vi "DoOperationDynamicDispatchMethod.vi"(8 "error in (no error)":errorcluster, 11 "SimpleArithmetic in":refnum<class "SimpleArithmetic.lvclass">) -> (0 "error out":errorcluster, 3 "SimpleArithmetic out":refnum<class "SimpleArithmetic.lvclass">)   [LabVIEW 2010, in "SimpleArithmetic.lvclass"]
uses:
  SimpleArithmetic.lvclass
  SimpleArithmetic.lvclass/SimpleArithmetic.ctl
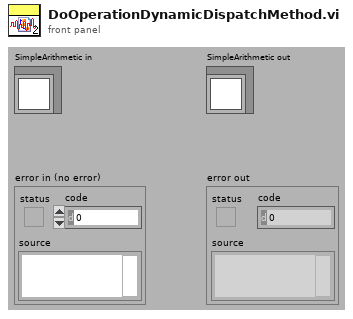
[diagram p1: front panel]
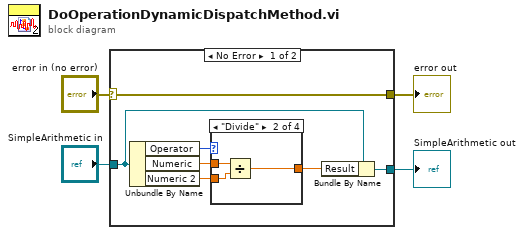
[diagram p0: block diagram]
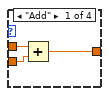
[diagram p2: hidden frame]
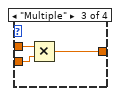
[diagram p3: hidden frame]
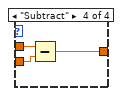
[diagram p4: hidden frame]
diagram:
  n1 = case shown="No Error" "error in (no error)" {
    selector: "error in (no error)" -> [w11 w25]
    tunnel: [w11 w25] -> w3
    tunnel: [w8 w24] -> w1
    tunnel: "SimpleArithmetic in" -> [w9 w24]
    frame No Error {
      n2 = Unbundle By Name(w9) -> ("Operator"=w10:enum16{"Add", "Divide", "Multiple", "Subtract"}, "Numeric"=w7:dbl, "Numeric 2"=w6:dbl)
      n3 = case shown="\"Divide\"" w10 {
        tunnel: w7 -> [w12 w17 w19 w22]
        tunnel: w6 -> [w13 w16 w20 w21]
        tunnel: [w14 w15 w18 w23] -> w5
        frame "Add" {
          n4 = Add(x=w12, y=w13) -> (x+y=w14:dbl)
        }
        frame "Divide" {
          n5 = Divide(x=w17, y=w16) -> (x/y=w15:dbl)
        }
        frame "Multiple" {
          n6 = Multiply(x=w19, y=w20) -> (x*y=w18:dbl)
        }
        frame "Subtract" {
          n7 = Subtract(x=w22, y=w21) -> (x-y=w23:dbl)
        }
      }
      n8 = Bundle By Name(cluster=w9, "Result"=w5) -> (w8:refnum<class "SimpleArithmetic.lvclass">)
    }
    frame Error {
    }
  }
  "error out" <- w3
  "SimpleArithmetic out" <- w1
